vi "Is Red Pitaya.vi"(8 "Error In":errorcluster, 9 "Acceptable logic tags":u16[](array[numeric])=[101, 102, 104, 109, 113, 159, 157, 152], 10 "Timeout":i32=100, 11 "Server address":string="192.168.1.100") -> (0 "Error Out":errorcluster, 1 "Status response":u32=1 format="0x%x (%d)", 2 "IDN response":u32=1 format="0x%x (%d)", 3 "Red Pitaya":bool, 4 "Error cleared?":bool, 5 "Logic tag out":u16, 6 "Module":i32, 7 "DDS modulus":i64)   [LabVIEW 2024, in "RP Communicator.lvclass"]
uses:
  RP Communicator.lvclass
  RP Communicator.lvclass/RP Communicator.ctl
  <vilib>/ErrorRing/Error Ring.xnode
  <vilib>/Utility/error.llb/Error Cluster From Error Code.vi
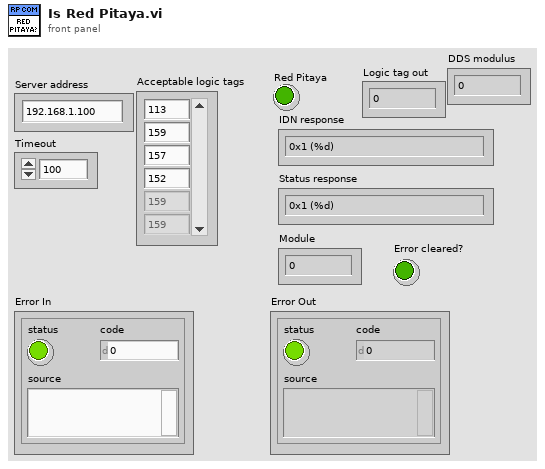
[diagram p1: front panel]
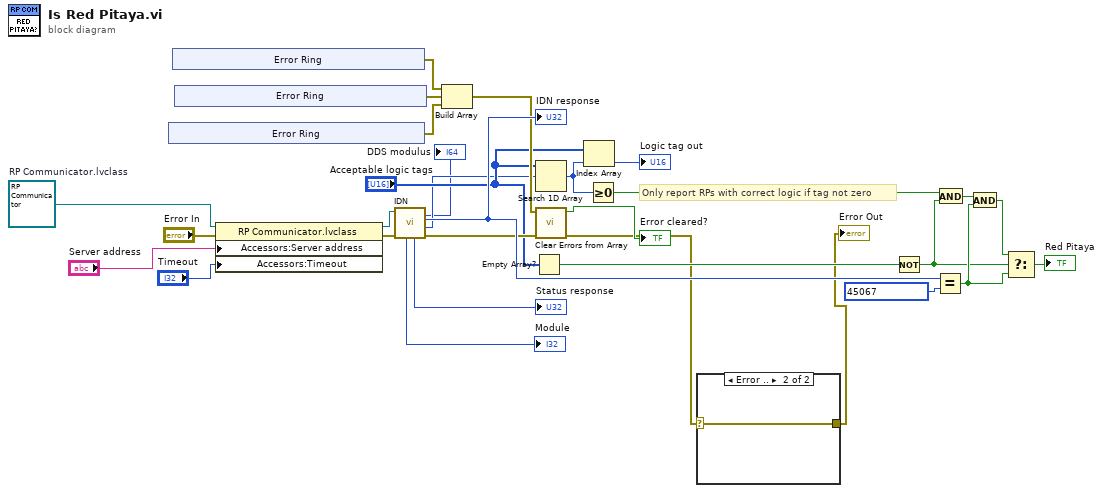
[diagram p0: block diagram]
diagram:
  w30 = refnum<class "RP Communicator.lvclass"> refnum  # RP Communicator.lvclass
  # "Only report RPs with correct logic if tag not zero"
  n1 = xnode "Error Ring"() -> ("error out"=w16:errorcluster)
  n2 = xnode "Error Ring"() -> ("error out"=w15:errorcluster)
  n3 = xnode "Error Ring"() -> ("error out"=w17:errorcluster)
  n4 = property class="RP Communicator.lvclass"(reference=w30, error in="Error In", "Accessors:Server address"="Server address", "Accessors:Timeout"="Timeout") -> (reference out=w27:refnum<class "RP Communicator.lvclass">, error out=w26:errorcluster)
  n5 = call-dynamic "IDN.vi"("error in (no error)"=w26, "RP Communicator in"=w27) -> ("error out"=w18:errorcluster, "Logic tag"=w4:u16, "IDN response"=w22:u32, "Status response"=→"Status response":u32, "DDS modulus"=→"DDS modulus":i64, "Module"=→"Module":i32)  [unwired: 3 in, 1 out]
  "IDN response" <- w22
  n6 = Build Array(w15, w17, w16) -> (w14:errorcluster[])
  n7 = Empty Array?(array="Acceptable logic tags") -> (empty?=w10:bool)
  n8 = Search 1D Array(1D array="Acceptable logic tags", element=w4) -> (index of element=w8:i32)  [unwired: 1 in]
  n9 = call "Clear Errors from Array.vi"("Error In"=w18, "Errors to clear"=w14) -> ("Error Out"=w2:errorcluster, "specific error cleared?"=→"Error cleared?":bool)  [unwired: 8 in]
  n10 = Index Array(array="Acceptable logic tags", index=w8) -> (element=→"Logic tag out":u16)
  n11 = Greater Or Equal To 0?(x=w8) -> (x >= 0?=w7:bool)
  n12 = case shown="Error .." w2 {
    selector: w2 -> [w31 w32]
    tunnel: [w31 w32] -> w1
    frame No Error {
    }
    frame Error {
    }
  }
  "Error Out" <- w1
  n13 = Not(x=w10) -> (.not. x?=w9:bool)
  n14 = Equal?(x=w22, y=u32 45067 ("IDN response")) -> (x = y?=w20:bool)
  n15 = And(x=w7, y=w9) -> (x .and. y?=w19:bool)
  n16 = And(x=w19, y=w20) -> (x .and. y?=w21:bool)
  n17 = Select(t=w21, s=w9, f=w20) -> (s? t:f=→"Red Pitaya":bool)
